vi "Warning Display.vi"(8 "error in (no error)":errorcluster) -> (0 "error out":errorcluster)   [LabVIEW 2020, in "Run Utilities.lvlib" / "Schedule Block.lvclass"]
uses:
  Schedule Block.lvclass
  Schedule Block.lvclass/Schedule Block.ctl
  TALOS.lvlib
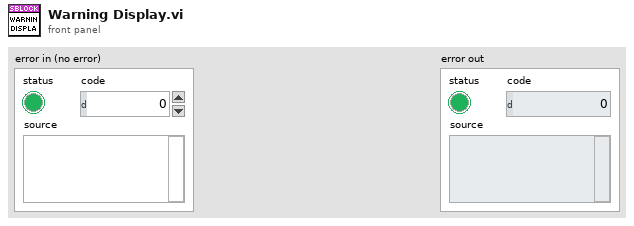
[diagram p1: front panel]
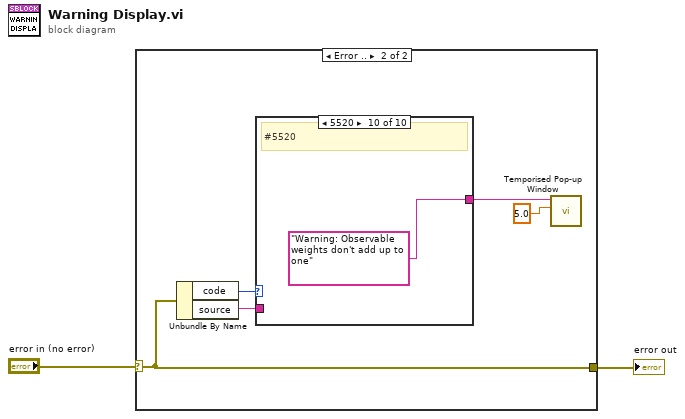
[diagram p0: block diagram]
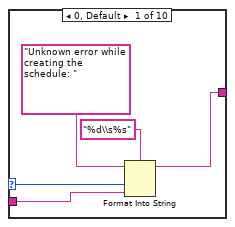
[diagram p3: hidden frame]
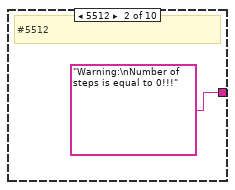
[diagram p4: hidden frame]
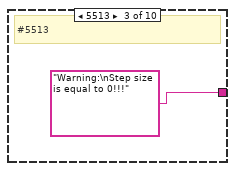
[diagram p5: hidden frame]
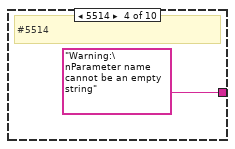
[diagram p6: hidden frame]
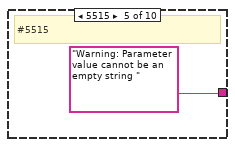
[diagram p7: hidden frame]
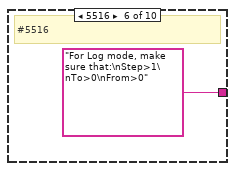
[diagram p8: hidden frame]
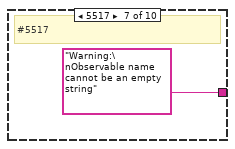
[diagram p9: hidden frame]
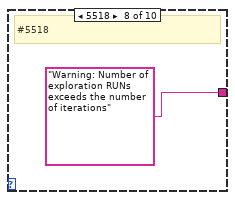
[diagram p10: hidden frame]
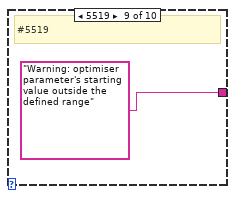
[diagram p11: hidden frame]
diagram:
  n1 = case shown="Error .." "error in (no error)" {
    selector: "error in (no error)" -> [w3 w4]
    tunnel: [w3 w4] -> w1
    frame No Error {
    }
    frame Error {
      n2 = Unbundle By Name(w4) -> ("code"=w6:i32, "source"=w5:string)
      n3 = case shown="5520" w6 {
        selector: w6 -> [w10 _ _ _ _ _ _ _ _ _]
        tunnel: [w11 "Warning:\nNumber of steps is equal to 0!!!" ("Text") "Warning:\nStep size is equal to 0!!!" ("source") "Warning:\nParameter name cannot be an empty string" ("source") "Warning: Parameter value cannot be an empty string " ("source") "For Log mode, make sure that:\nStep>1\nTo>0\nFrom>0" ("source") "Warning:\nObservable name cannot be an empty string" ("source") "Warning: Number of exploration RUNs exceeds the number of iterations" ("Text") "Warning: optimiser parameter's starting value outside the defined range" ("Text") "Warning: Observable weights don't add up to one" ("source")] -> w7
        tunnel: w5 -> [w9 _ _ _ _ _ _ _ _ _]
        frame 0, Default {
          n4 = Format Into String(format string="%d\\s%s", initial string="Unknown error while creating the schedule: " ("Text"), w10, w9) -> (resulting string=w11:string)  [unwired: 1 in, 1 out]
        }
        frame 5512 {
          # "#5512"
        }
        frame 5513 {
          # "#5513"
        }
        frame 5514 {
          # "#5514"
        }
        frame 5515 {
          # "#5515"
        }
        frame 5516 {
          # "#5516"
        }
        frame 5517 {
          # "#5517"
        }
        frame 5518 {
          # "#5518"
        }
        frame 5519 {
          # "#5519"
        }
        frame 5520 {
          # "#5520"
        }
      }
      n5 = call "Temporised Pop-up Window.vi"("Timeout"=5.0, "Text"=w7) -> ()  [unwired: 9 in, 1 out]
    }
  }
  "error out" <- w1
